vi "Translator.vi"(8 "error in (no error)":errorcluster, 11 "Input":variant) -> (0 "error out":errorcluster, 3 "Output":variant)   [LabVIEW 2014, in "Arduino MPU6050.lvlib"]
doc: "An example of how to create the Translator to convert the LabVIEW VIs to Arduino C code."
uses:
  Arduino MPU6050.lvlib
panel:
  out "Outputs":string[](array[string])
  out "Inputs":string[](array[string])
  out "Output Datatypes":string[](array[string])
  out "Input Datatypes":string[](array[string])
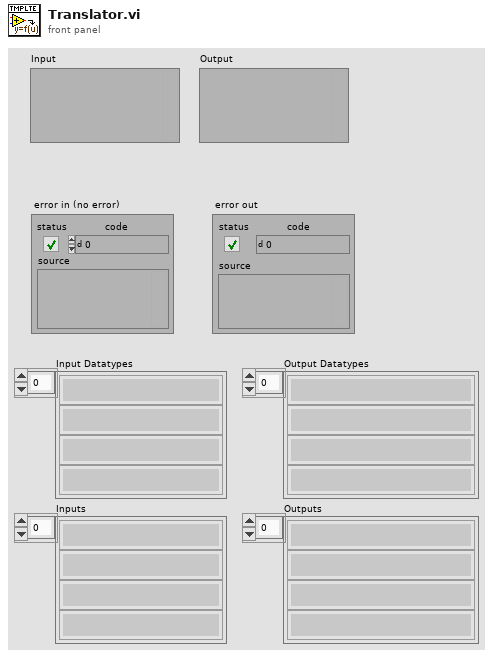
[diagram p1: front panel]
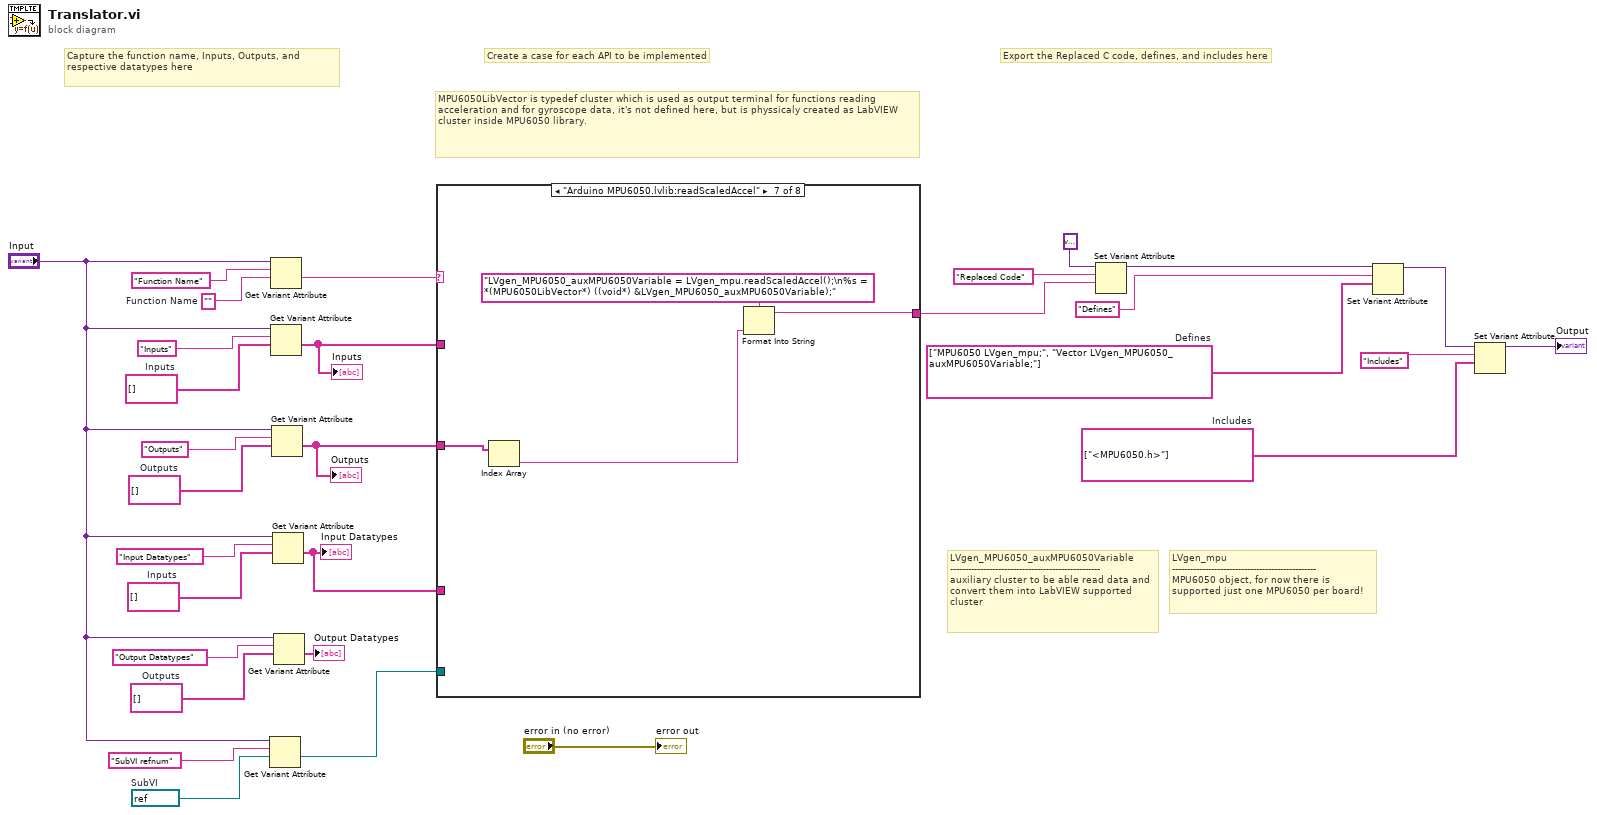
[diagram p0: block diagram]
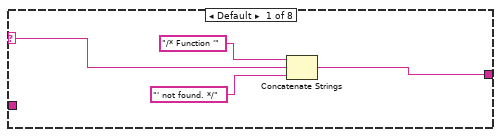
[diagram p2: hidden frame]
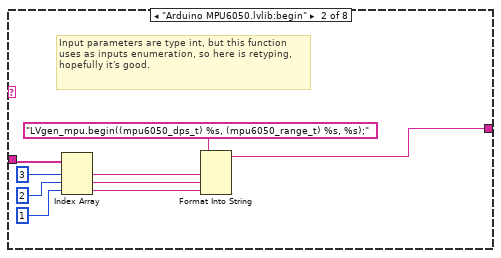
[diagram p3: hidden frame]
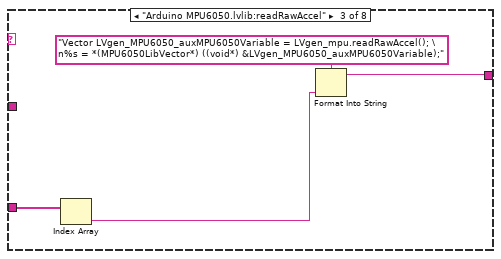
[diagram p4: hidden frame]
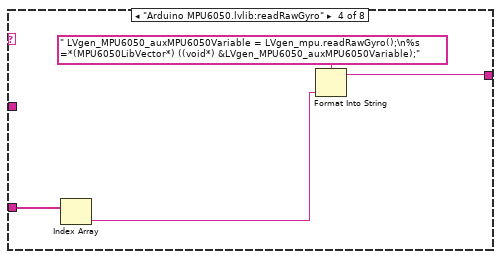
[diagram p5: hidden frame]
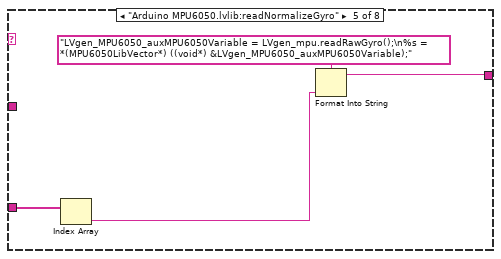
[diagram p6: hidden frame]
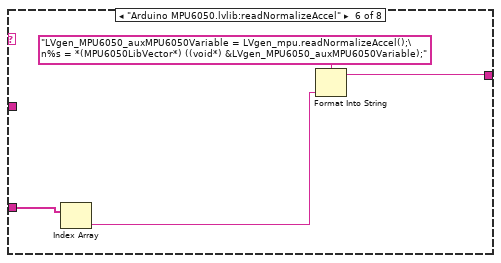
[diagram p7: hidden frame]
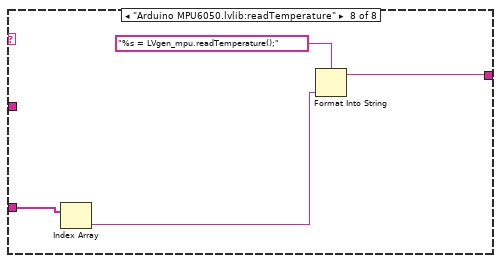
[diagram p8: hidden frame]
diagram:
  w2 = refnum<vi> refnum  # SubVI
  w6 = string[] ["MPU6050 LVgen_mpu;", "Vector LVgen_MPU6050_auxMPU6050Variable;"]  # Defines
  w15 = string[] []  # Outputs
  w16 = string[] []  # Inputs
  w21 = string[] ["<MPU6050.h>"]  # Includes
  w26 = string[] []  # Outputs
  w27 = string[] []  # Inputs
  w28 = ""  # Function Name
  # "MPU6050LibVector is typedef cluster which is used as output terminal for functions reading acceleration and for gyroscope data, it's not defined here, but is physsicaly created as LabVIEW cluster inside MPU6050 library."
  # "LVgen_MPU6050_auxMPU6050Variable\n--------------------------------------------------\nauxiliary cluster to be able read data and convert them into LabVIEW supported cluster"
  # "LVgen_mpu\n------------------------------------------------\nMPU6050 object, for now there is supported just one MPU6050 per board!"
  # "Capture the function name, Inputs, Outputs, and respective datatypes here"
  # "Export the Replaced C code, defines, and includes here"
  # "Create a case for each API to be implemented"
  n1 = Get Variant Attribute(Variant="Input", name="SubVI refnum", default value (empty Variant)=w2) -> (value=w1:refnum<vi>)  [unwired: 1 in, 3 out]
  n2 = Get Variant Attribute(Variant="Input", name="Function Name", default value (empty Variant)=w28) -> (value=w23:string)  [unwired: 1 in, 3 out]
  n3 = Get Variant Attribute(Variant="Input", name="Inputs", default value (empty Variant)=w27) -> (value=w11:string[])  [unwired: 1 in, 3 out]
  "Inputs" <- w11
  n4 = Get Variant Attribute(Variant="Input", name="Outputs", default value (empty Variant)=w26) -> (value=w12:string[])  [unwired: 1 in, 3 out]
  "Outputs" <- w12
  n5 = Get Variant Attribute(Variant="Input", name="Input Datatypes", default value (empty Variant)=w16) -> (value=w5:string[])  [unwired: 1 in, 3 out]
  "Input Datatypes" <- w5
  n6 = Get Variant Attribute(Variant="Input", name="Output Datatypes", default value (empty Variant)=w15) -> (value=→"Output Datatypes":string[])  [unwired: 1 in, 3 out]
  n7 = case shown="\"Arduino MPU6050.lvlib:readScaledAccel\"" w23 {
    selector: w23 -> [w33 _ _ _ _ _ _ _]
    tunnel: [w31 w35 w46 w50 w54 w58 w62 w66] -> w22
    tunnel: w11 -> [_ w42 _ _ _ _ _ _]
    tunnel: w12 -> [_ _ w47 w51 w55 w59 w63 w67]
    tunnel: w5 -> [_ _ _ _ _ _ _ _]
    tunnel: w1 -> [_ _ _ _ _ _ _ _]
    frame Default {
      n8 = Concatenate Strings("/* Function '", w33, "' not found. */") -> (w31:string)
    }
    frame "Arduino MPU6050.lvlib:begin" {
      # "Input parameters are type int, but this function uses as inputs enumeration, so here is retyping, hopefully it's good."
      n9 = Index Array(array=w42, index #1=3 ("index"), index #2=2 ("index"), index #3=1 ("index")) -> (element #1=w38:string, element #2=w37:string, element #3=w36:string)
      n10 = Format Into String(format string="LVgen_mpu.begin((mpu6050_dps_t) %s, (mpu6050_range_t) %s, %s);", w38, w37, w36) -> (resulting string=w35:string)  [unwired: 2 in, 1 out]
    }
    frame "Arduino MPU6050.lvlib:readRawAccel" {
      n11 = Index Array(array=w47) -> (element=w44:string)  [unwired: 1 in]
      n12 = Format Into String(format string="Vector LVgen_MPU6050_auxMPU6050Variable = LVgen_mpu.readRawAccel(); \n%s = *(MPU6050LibVector*) ((void*) &LVgen_MPU6050_auxMPU6050Variable);", w44) -> (resulting string=w46:string)  [unwired: 2 in, 1 out]
    }
    frame "Arduino MPU6050.lvlib:readRawGyro" {
      n13 = Index Array(array=w51) -> (element=w48:string)  [unwired: 1 in]
      n14 = Format Into String(format string=" LVgen_MPU6050_auxMPU6050Variable = LVgen_mpu.readRawGyro();\n%s =*(MPU6050LibVector*) ((void*) &LVgen_MPU6050_auxMPU6050Variable);", w48) -> (resulting string=w50:string)  [unwired: 2 in, 1 out]
    }
    frame "Arduino MPU6050.lvlib:readNormalizeGyro" {
      n15 = Index Array(array=w55) -> (element=w52:string)  [unwired: 1 in]
      n16 = Format Into String(format string="LVgen_MPU6050_auxMPU6050Variable = LVgen_mpu.readRawGyro();\n%s = *(MPU6050LibVector*) ((void*) &LVgen_MPU6050_auxMPU6050Variable);", w52) -> (resulting string=w54:string)  [unwired: 2 in, 1 out]
    }
    frame "Arduino MPU6050.lvlib:readNormalizeAccel" {
      n17 = Index Array(array=w59) -> (element=w56:string)  [unwired: 1 in]
      n18 = Format Into String(format string="LVgen_MPU6050_auxMPU6050Variable = LVgen_mpu.readNormalizeAccel();\n%s = *(MPU6050LibVector*) ((void*) &LVgen_MPU6050_auxMPU6050Variable);", w56) -> (resulting string=w58:string)  [unwired: 2 in, 1 out]
    }
    frame "Arduino MPU6050.lvlib:readScaledAccel" {
      n19 = Index Array(array=w63) -> (element=w60:string)  [unwired: 1 in]
      n20 = Format Into String(format string="LVgen_MPU6050_auxMPU6050Variable = LVgen_mpu.readScaledAccel();\n%s = *(MPU6050LibVector*) ((void*) &LVgen_MPU6050_auxMPU6050Variable);", w60) -> (resulting string=w62:string)  [unwired: 2 in, 1 out]
    }
    frame "Arduino MPU6050.lvlib:readTemperature" {
      n21 = Index Array(array=w67) -> (element=w64:string)  [unwired: 1 in]
      n22 = Format Into String(format string="%s = LVgen_mpu.readTemperature();", w64) -> (resulting string=w66:string)  [unwired: 2 in, 1 out]
    }
  }
  n23 = Set Variant Attribute(Variant=variant ("variant"), name="Replaced Code", value=w22) -> (Variant out=w9:variant)  [unwired: 1 in, 2 out]
  n24 = Set Variant Attribute(Variant=w9, name="Defines", value=w6) -> (Variant out=w8:variant)  [unwired: 1 in, 2 out]
  n25 = Set Variant Attribute(Variant=w8, name="Includes", value=w21) -> (Variant out=→"Output":variant)  [unwired: 1 in, 2 out]
  "error out" <- "error in (no error)"
